vi "回零.vi"(10 "Change Value":dbl=10.0, 11 "AxisHandle IN":u32) -> (3 "AxisHandle OUT":u32)   [LabVIEW 2013]
panel:
  out "error out":errorcluster
  out "ReturnValue":u32
  out "输出变量":dbl
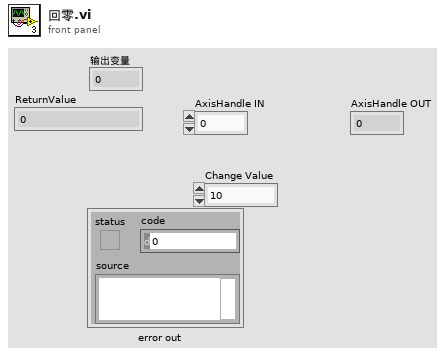
[diagram p1: front panel]
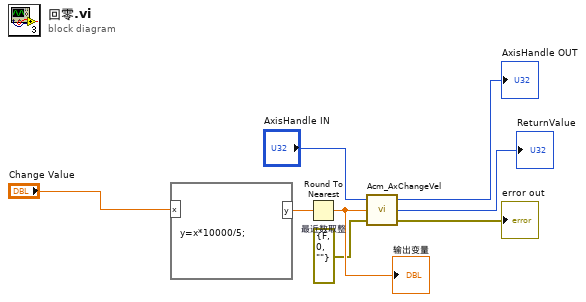
[diagram p0: block diagram]
diagram:
  n1 = formula code="y=x*10000/5;"("x"="Change Value") -> ("y"=w1:dbl)
  n2 = Round To Nearest "最近数取整"(number=w1) -> (nearest integer value=w4:dbl)
  "输出变量" <- w4
  n3 = call <userlib>:"Acm_AxChangeVel.vi"("Error Input(No Error)"=errorcluster {"status"=FALSE, "code"=0, "source"=""}, "NewVelocity"=w4, "AxisHandle"="AxisHandle IN") -> ("Error Output"=→"error out":errorcluster, "ReturnValue"=→"ReturnValue":u32, "AxisHandle 2"=→"AxisHandle OUT":u32)
